vi "outliers.vi"(0 "U2":dbl format="%.2f", 1 "U1":dbl format="%.2f", 2 "L1":dbl format="%.2f", 3 "L2":dbl format="%.2f", 4 "Raw Data":dbl[](array[numeric]) format="%.2f") -> (5 "Far Outliers":dbl[](array[numeric]) format="%.2f", 6 "Near Outliers":dbl[](array[numeric]) format="%.2f")   [LabVIEW 2021, in "statistics.lvlib"]
uses:
  statistics.lvlib
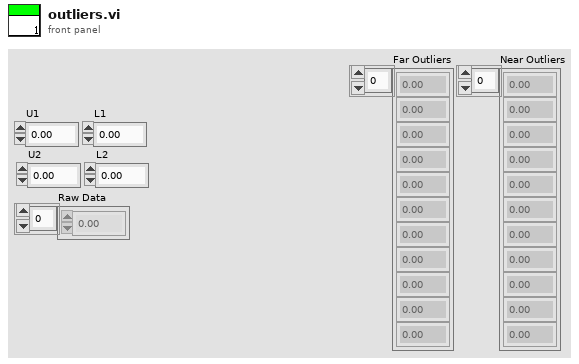
[diagram p1: front panel]
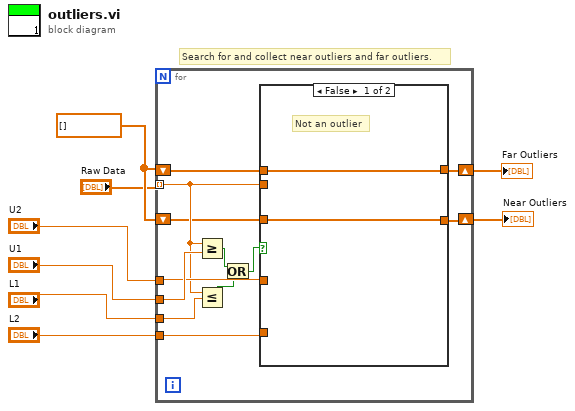
[diagram p0: block diagram]
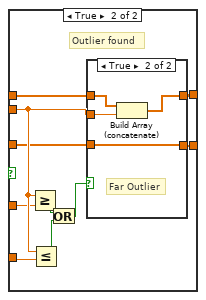
[diagram p2: hidden frame]
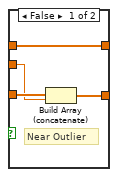
[diagram p3: hidden frame]
diagram:
  w2 = dbl[] []
  # "Search for and collect near outliers and far outliers."
  n1 = for {
    tunnel: "Raw Data" -> [w17] mode=indexing
    shift-right: [w11] -> w4
    shift-left: w2 -> [w18]
    shift-right: [w9] -> w3
    shift-left: w2 -> [w10]
    tunnel: "U2" -> [w19]
    tunnel: "U1" -> [w20]
    tunnel: "L1" -> [w16]
    tunnel: "L2" -> [w12]
    n2 = Greater Or Equal?(x=w17, y=w20) -> (x >= y?=w14:bool)
    n3 = Less Or Equal?(x=w17, y=w16) -> (x <= y?=w15:bool)
    n4 = Or(x=w14, y=w15) -> (x .or. y?=w13:bool)
    n5 = case shown="False" w13 {
      tunnel: w17 -> [_ w30]
      tunnel: w19 -> [_ w29]
      tunnel: w18 -> [w22 w25]
      tunnel: w12 -> [_ w28]
      tunnel: [w22 w32] -> w11
      tunnel: w10 -> [w21 w24]
      tunnel: [w21 w23] -> w9
      frame False {
        # "Not an outlier"
      }
      frame True {
        # "Outlier found"
        n6 = Greater Or Equal?(x=w30, y=w29) -> (x >= y?=w27:bool)
        n7 = Less Or Equal?(x=w30, y=w28) -> (x <= y?=w26:bool)
        n8 = Or(x=w27, y=w26) -> (x .or. y?=w31:bool)
        n9 = case shown="True" w31 {
          tunnel: [w36 w38] -> w32
          tunnel: w30 -> [w34 w40]
          tunnel: w25 -> [w36 w39]
          tunnel: w24 -> [w35 w37]
          tunnel: [w33 w37] -> w23
          frame False {
            # "Near Outlier"
            n10 = Build Array (concatenate)(w35, w34) -> (w33:dbl[])
          }
          frame True {
            # "Far Outlier"
            n11 = Build Array (concatenate)(w39, w40) -> (w38:dbl[])
          }
        }
      }
    }
  }
  "Far Outliers" <- w4
  "Near Outliers" <- w3
